vi "sv_Traditional DAQ Prefix.vi"() -> (0 "Traditional DAQ prefix":string="$_SVT Swept Sine Task Traditional DAQ_$ : ")   [LabVIEW 2017, in "SoundVib_SweptSine.lvlib"]
uses:
  <vilib>/addons/Sound and Vibration/svt_Swept Sine/SoundVib_SweptSine.lvlib
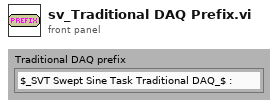
[diagram p1: front panel]
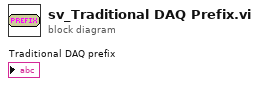
[diagram p0: block diagram]
diagram:
